vi "TESTE CURVA GRUPO-2.vi"() -> ()   [LabVIEW 2014]
uses:
  <userlib>/Newport ESP301/Newport ESP301.lvlib
panel:
  in  "Raio":dbl=100.0
  out "Yin":dbl format="%.6g"
  out "Xin":dbl format="%.6g"
  out "d (um)":dbl
  in  "d":dbl=100.0
  in  "Velocity":dbl=1.0
  # "tamanho da amostra (mm)"
  # "distancia entrada saída (um)"
  # "Inicio curva"
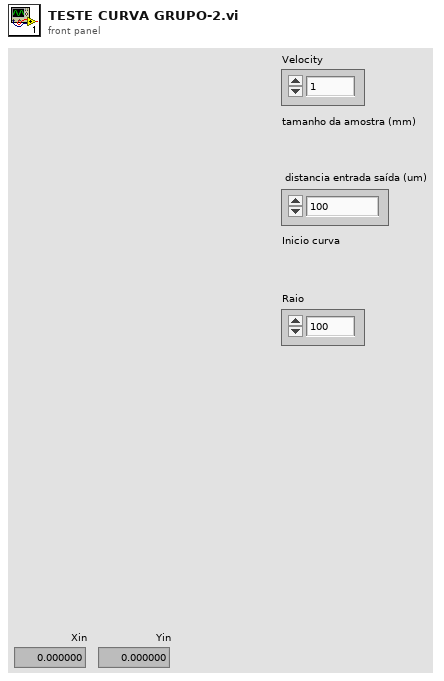
[diagram p1: front panel]
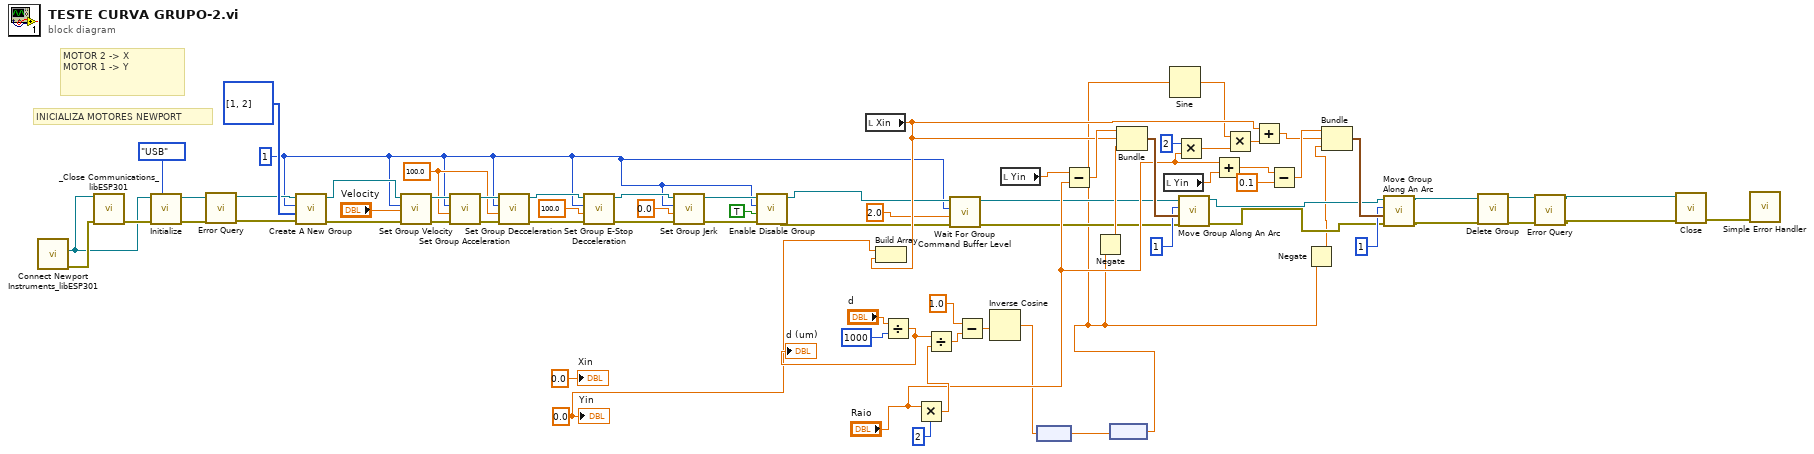
[diagram p0: block diagram]
diagram:
  w32 = 0.0 ("Yin")
  w10 = 1 ("Group #")
  w61 = 100.0 ("Acceleration (0 units/s²)")
  # "MOTOR 2 -> X\nMOTOR 1 -> Y"
  # "INICIALIZA MOTORES NEWPORT"
  n1 = call <userlib>:"Connect Newport Instruments_libESP301.vi"() -> ("error (duplicate)"=w71:errorcluster, "VISA resource name (duplicate)"=w70:refnum<visa-resource-name>)  [unwired: 7 in, 3 out]
  n2 = call <userlib>:"_Close Communications_libESP301.vi"("Instrument Channel"=w70, "error in (no error)"=w71) -> ("error out"=w73:errorcluster)  [unwired: 13 in]
  n3 = call <userlib>:"Initialize.vi"("VISA resource name"=w70, "error in (no error)"=w73, "Serial Link (RS232)"=enum16{"RS232", "USB"}."USB") -> ("VISA resource name out"=w51:refnum<visa-resource-name>, "error out"=w50:errorcluster)  [unwired: 6 in]
  n4 = call <userlib>:"Error Query.vi"("error in (no error)"=w50, "VISA resource name"=w51) -> ("error out"=w48:errorcluster, "VISA resource name out"=w49:refnum<visa-resource-name>)  [unwired: 2 in, 2 out]
  n5 = call <userlib>:"Create A New Group.vi"("error in (no error)"=w48, "Axis Number"=i32[] [1, 2], "Group Number (1)"=w10, "VISA resource name"=w49) -> ("error out"=w67:errorcluster, "VISA resource name out"=w68:refnum<visa-resource-name>)  [unwired: 2 in]
  n6 = call <userlib>:"Set Group Velocity.vi"("error in (no error)"=w67, "Velocity (units/s)"="Velocity", "Group Number (1)"=w10, "VISA resource name"=w68) -> ("error out"=w62:errorcluster, "VISA resource name out"=w65:refnum<visa-resource-name>)  [unwired: 2 in]
  n7 = call <userlib>:"Set Group Acceleration.vi"("error in (no error)"=w62, "Acceleration (0 units/s²)"=w61, "Group Number (1)"=w10, "VISA resource name"=w65) -> ("error out"=w63:errorcluster, "VISA resource name out"=w64:refnum<visa-resource-name>)  [unwired: 2 in]
  n8 = call <userlib>:"Set Group Decceleration.vi"("error in (no error)"=w63, "Decceleration (0 units/s²)"=w61, "Group Number (1)"=w10, "VISA resource name"=w64) -> ("error out"=w57:errorcluster, "VISA resource name out"=w60:refnum<visa-resource-name>)  [unwired: 2 in]
  n9 = call <userlib>:"Set Group E-Stop Decceleration.vi"("error in (no error)"=w57, "E-Stop Decceleration (0 units/s²)"=100.0, "Group Number (1)"=w10, "VISA resource name"=w60) -> ("error out"=w56:errorcluster, "VISA resource name out"=w59:refnum<visa-resource-name>)  [unwired: 2 in]
  n10 = call <userlib>:"Set Group Jerk.vi"("error in (no error)"=w56, "Vector Jerk (0 units/s^3)"=0.0, "Group Number (1)"=w10, "VISA resource name"=w59) -> ("error out"=w55:errorcluster, "VISA resource name out"=w58:refnum<visa-resource-name>)  [unwired: 2 in]
  n11 = call <userlib>:"Enable Disable Group.vi"("error in (no error)"=w55, "Action (OFF)"=TRUE, "Group Number (1)"=w10, "VISA resource name"=w58) -> ("error out"=w16:errorcluster, "VISA resource name out"=w17:refnum<visa-resource-name>)  [unwired: 2 in]
  n12 = local read "Xin"() -> (w27:dbl)
  n13 = Build Array(w32, w27) -> ()  [unwired: 1 out]
  n14 = Divide(x="d", y=1000) -> (x/y=w34:dbl)
  "d (um)" <- w34
  n15 = Multiply(x="Raio", y=2) -> (x*y=w46:dbl)
  n16 = Divide(x=w34, y=w46) -> (x/y=w23:dbl)
  n17 = call <userlib>:"Wait For Group Command Buffer Level.vi"("error in (no error)"=w16, "level in group via point buffer"=2.0, "Group Number (1)"=w10, "VISA resource name"=w17) -> ("error out"=w14:errorcluster, "VISA resource name out"=w15:refnum<visa-resource-name>)  [unwired: 2 in]
  n18 = Subtract(x=1.0, y=w23) -> (x-y=w21:dbl)
  n19 = Inverse Cosine(1:w21) -> (0:w8:dbl)
  n20 = local read "Yin"() -> (w30:dbl)
  n21 = node(w8) -> (w9:dbl[unit])
  n22 = Subtract(x=w30, y="Raio") -> (x-y=w45:dbl)
  n23 = node(w9) -> (w7:dbl)
  n24 = Negate(x=w7) -> (-x=w20:dbl)
  n25 = Bundle(w45, "Xin"=w27, w20) -> (w44:cluster{dbl, "Xin":dbl, dbl})  [unwired: 1 in]
  n26 = local read "Yin"() -> (w39:dbl)
  n27 = Sine(x=w7) -> (sin(x)=w26:dbl)
  n28 = Multiply(x=2, y="Raio") -> (x*y=w25:dbl)
  n29 = call <userlib>:"Move Group Along An Arc.vi"("error in (no error)"=w14, "Arc  Parameters"=w44, "Group Number (1)"=1, "VISA resource name"=w15) -> ("error out"=w12:errorcluster, "VISA resource name out"=w13:refnum<visa-resource-name>)  [unwired: 2 in]
  n30 = Add(x="Raio", y=w39) -> (x+y=w40:dbl)
  n31 = Multiply(x=w26, y=w25) -> (x*y=w24:dbl)
  n32 = Add(x=w27, y=w24) -> (x+y=w37:dbl)
  n33 = Subtract(x=w40, y=0.1) -> (x-y=w43:dbl)
  n34 = Negate(x=w7) -> (-x=w2:dbl)
  n35 = Bundle(w43, w37, w2) -> (w42:cluster{dbl, dbl, dbl})  [unwired: 1 in]
  n36 = call <userlib>:"Move Group Along An Arc.vi"("error in (no error)"=w12, "Arc  Parameters"=w42, "Group Number (1)"=1, "VISA resource name"=w13) -> ("error out"=w18:errorcluster, "VISA resource name out"=w19:refnum<visa-resource-name>)  [unwired: 2 in]
  n37 = call <userlib>:"Delete Group.vi"("error in (no error)"=w18, "VISA resource name"=w19) -> ("error out"=w5:errorcluster, "VISA resource name out"=w6:refnum<visa-resource-name>)  [unwired: 4 in]
  n38 = call <userlib>:"Error Query.vi"("error in (no error)"=w5, "VISA resource name"=w6) -> ("error out"=w3:errorcluster, "VISA resource name out"=w4:refnum<visa-resource-name>)  [unwired: 2 in, 2 out]
  n39 = call <userlib>:"Close.vi"("error in (no error)"=w3, "VISA resource name"=w4) -> ("error out"=w1:errorcluster)  [unwired: 9 in]
  n40 = call <vilib>:"Simple Error Handler.vi"("error in (no error)"=w1) -> ()  [unwired: 4 in, 5 out]
  "Xin" <- 0.0 ("Xin")
  "Yin" <- w32
